vi "put.vi"(7 "transmit queue":refnum<queue>, 10 "application request in":T1, 11 "http responder in":refnum<class "http responder.lvclass">) -> (0 "error out":errorcluster, 3 "http responder out":refnum<class "http responder.lvclass">)   [LabVIEW 2013, in "http responder.lvclass"]
uses:
  http responder.lvclass
  HTTP server/http response.ctl
  HTTP server/http response packet type.ctl
  HTTP headers/http header data.ctl
  HTTP server/http request.ctl
  HTTP server/http method.ctl
  URI/url structure.ctl
  HTTP server/Basic HTTP server.lvclass
  HTTP headers/http headers.lvlib
  URI/uniform resource locator.lvlib
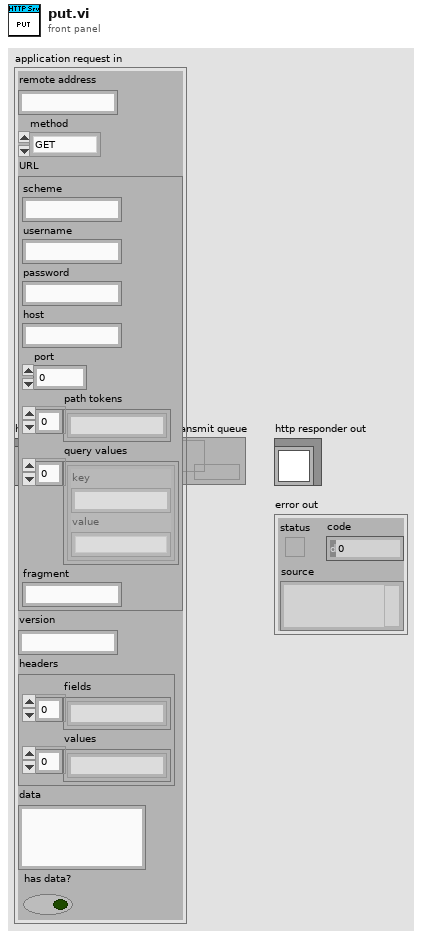
[diagram p1: front panel]
types:
  T1 = typedef "Basic HTTP server.lvclass/http request.ctl" = cluster{"remote address":string, "method":T2, "URL":T3, "version":string, "headers":T4, "data":string, "has data?":bool}
  T2 = typedef "Basic HTTP server.lvclass/http method.ctl" = enum16{"GET", "POST", "PUT", "DELETE", "HEAD", "OPTIONS", "upgrade"}
  T3 = typedef "uniform resource locator.lvlib/url structure.ctl" = cluster{"scheme":string, "username":string, "password":string, "host":string, "port":u16, "path tokens":string[], "query values":cluster{"key":string, "value":string}[], "fragment":string}
  T4 = typedef "http headers.lvlib/http header data.ctl" = cluster{"fields":string[], "values":string[]}
  T5 = typedef "Basic HTTP server.lvclass/http response packet type.ctl" = enum16{"full response", "header only", "data only", "last data"}
  T6 = typedef "Basic HTTP server.lvclass/http response.ctl" = cluster{"packet type":T5, "reason code":u16, "status string":string, "headers":T4, "cookies":string[], "data":string}
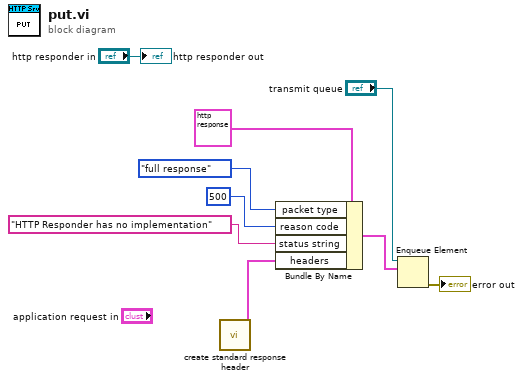
[diagram p0: block diagram]
diagram:
  n1 = call "create standard response header.vi"() -> ("default header"=w1:T4)  [unwired: 11 in]
  n2 = Bundle By Name(cluster=T6 {"packet type"=enum."full response", "reason code"=0, "status string"="", "headers"={"fields"=[], "values"=[]}, "cookies"=[], "data"=""} ("application request"), "packet type"=http_response_packet_type."full response", "reason code"=u16 500, "status string"="HTTP Responder has no implementation", "headers"=w1) -> (w8:T6)
  n3 = Enqueue Element(queue="transmit queue", element=w8) -> (error out=→"error out":errorcluster)  [unwired: 2 in, 2 out]
  "http responder out" <- "http responder in"
